vi "TimeCounter.vi"(10 "Limit [ms]":u32, 11 "Reset(T)/Count(F)":bool) -> (2 "Overlimit?":bool, 3 "Counter [ms]":u32)   [LabVIEW 2020]
panel:
  out "error out":errorcluster
  in  "error in (no error)":errorcluster
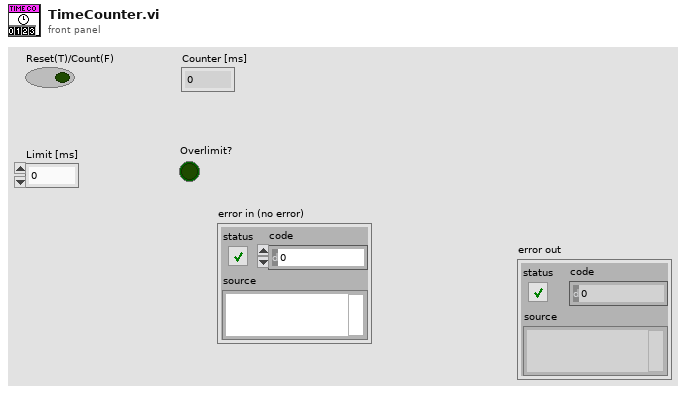
[diagram p1: front panel]
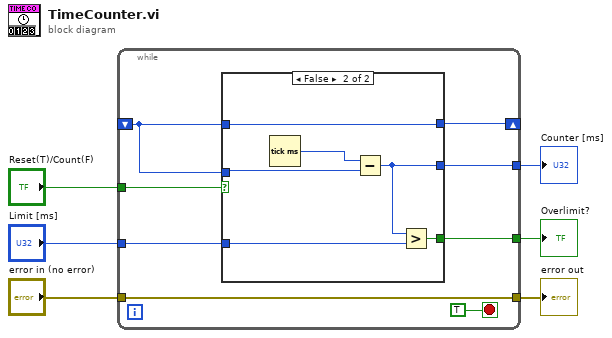
[diagram p0: block diagram]
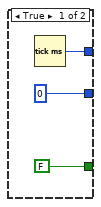
[diagram p2: hidden frame]
diagram:
  n1 = while {
    tunnel: "Reset(T)/Count(F)" -> [w13]
    shift-right: [w12] -> _
    shift-left: _ -> [w10]
    tunnel: [w11] -> w5
    tunnel: "Limit [ms]" -> [w9]
    tunnel: [w8] -> w6
    tunnel: "error in (no error)" -> [w7]
    tunnel: [w7] -> w1
    stop <- TRUE stop-if-true
    n2 = case shown="False" w13 {
      tunnel: w10 -> [_ w22]
      tunnel: [w17 w21] -> w12
      tunnel: [u32 0 w19] -> w11
      tunnel: w10 -> [_ w21]
      tunnel: w9 -> [_ w20]
      tunnel: [FALSE w18] -> w8
      frame True {
        n3 = Tick Count (ms)() -> (millisecond timer value=w17:u32)
      }
      frame False {
        n4 = Tick Count (ms)() -> (millisecond timer value=w23:u32)
        n5 = Subtract(x=w23, y=w22) -> (x-y=w19:u32)
        n6 = Greater?(x=w19, y=w20) -> (0:w18:bool)
      }
    }
  }
  "Counter [ms]" <- w5
  "Overlimit?" <- w6
  "error out" <- w1
